vi "Write Path.vi"(8 "error in (no error)":errorcluster, 10 "Path":path, 11 "Config_Read_SPI in":refnum<class "Config_Read_SPI.lvclass">) -> (0 "error out":errorcluster, 3 "Config_Read_SPI out":refnum<class "Config_Read_SPI.lvclass">)   [LabVIEW 2018, in "Config_Read_SPI.lvclass"]
uses:
  Config_Read_SPI.lvclass
  Config_Read_SPI.lvclass/Config_Read_SPI.ctl
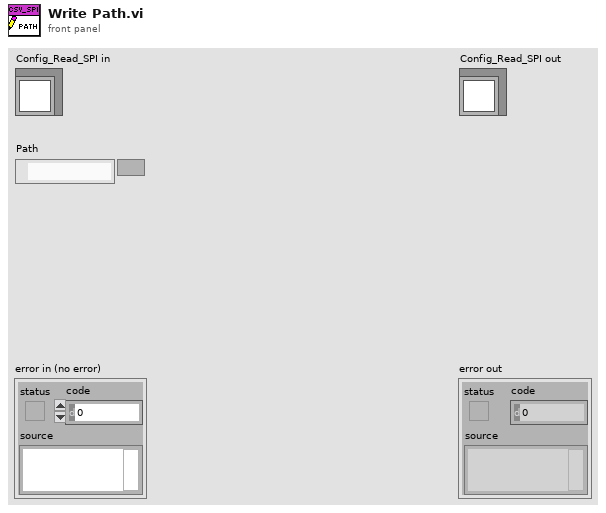
[diagram p1: front panel]
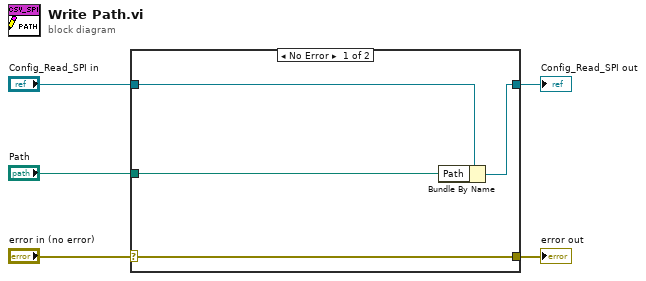
[diagram p0: block diagram]
diagram:
  n1 = case shown="No Error" "error in (no error)" {
    selector: "error in (no error)" -> [w9 w10]
    tunnel: [w9 w10] -> w4
    tunnel: [w7 w11] -> w2
    tunnel: "Config_Read_SPI in" -> [w8 w11]
    tunnel: "Path" -> [w6 _]
    frame No Error {
      n2 = Bundle By Name(cluster=w8, "Path"=w6) -> (w7:refnum<class "Config_Read_SPI.lvclass">)
    }
    frame Error {
    }
  }
  "error out" <- w4
  "Config_Read_SPI out" <- w2
